vi "sub_APT.vi"() -> ()   [LabVIEW 2015]
panel:
  in  "Up":bool
  in  "Abs. Go":bool
  in  "Down":bool
  in  "Rel Move Size":sgl=1.0 min=-10 max=50 format="%.2f"
  in  "Home Z":bool
  in  "Abs Pos X":sgl=1.0 min=-10 max=360 format="%.2f"
  out "Display Z":sgl(knob) scale=0.0..360.0
  out "Initial Z":bool
  in  "HWSerialNum Z":i32=83856379
  in  "Stop":bool
  in  "MG17Motor Z":refnum<k7>(container)
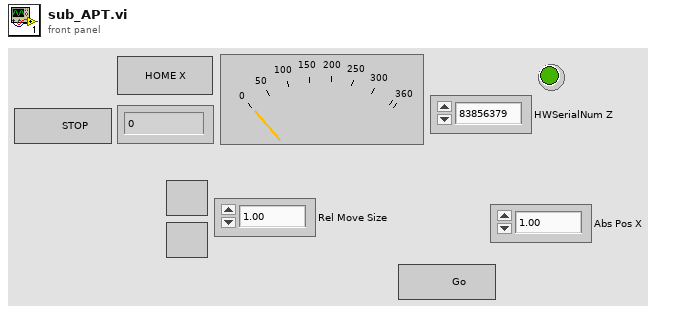
[diagram p1: front panel]
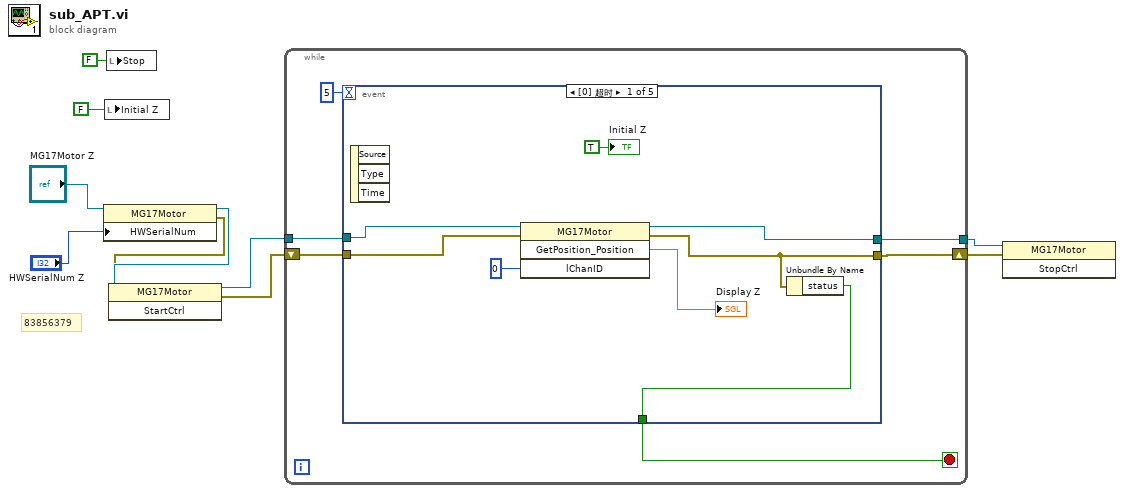
[diagram p0: block diagram]
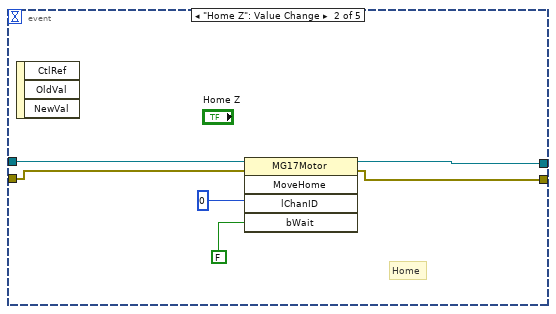
[diagram p2: hidden frame]
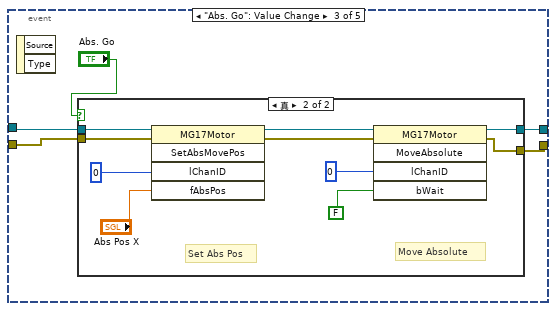
[diagram p3: hidden frame]
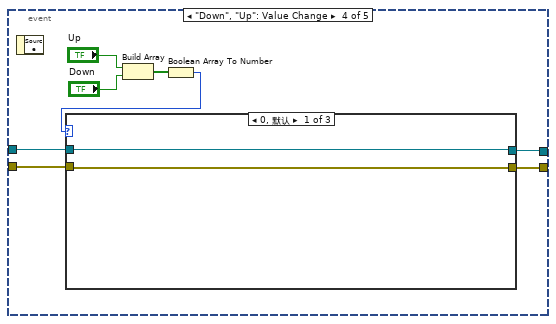
[diagram p5: hidden frame]
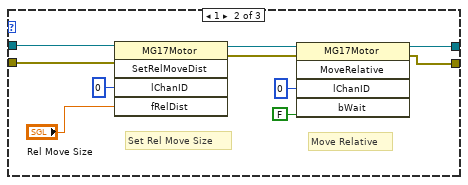
[diagram p6: hidden frame]
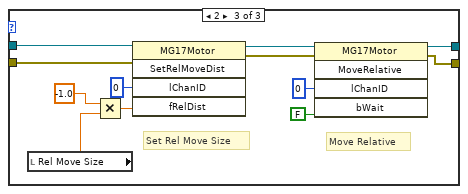
[diagram p7: hidden frame]
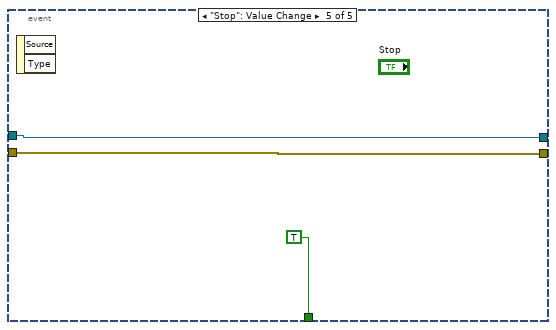
[diagram p8: hidden frame]
diagram:
  # "83856379"
  n1 = property class="MG17Motor"(reference="MG17Motor Z", "HWSerialNum"="HWSerialNum Z") -> (reference out=w9:refnum<k7>, error out=w8:errorcluster)  [unwired: 1 in]
  n2 = local write "Initial Z"(FALSE ("Initial")) -> ()
  n3 = local write "Stop"(FALSE ("Stop")) -> ()
  n4 = invoke class="MG17Motor" method="StartCtrl"(reference=w9, error in=w8) -> (reference out=w7:refnum<k7>, error out=w6:errorcluster)  [unwired: 1 in, 1 out]
  n5 = while {
    shift-right: [w13] -> w4
    shift-left: w6 -> [w15]
    tunnel: w7 -> [w16]
    tunnel: [w14] -> w5
    stop <- w11 stop-if-true
    n6 = event shown="[0] 超时" {
      selector: _ -> [_ _ _ _ _]
      dyn-events: _ -> [_ _ _ _ _]
      timeout: 5 -> [_ _ _ _ _]
      tunnel: w16 -> [w23 w28 w35 w55 w81]
      tunnel: w15 -> [w21 w27 w34 w54 w80]
      tunnel: [w22 w26 w33 w53 w81] -> w14
      tunnel: [w18 w25 w32 w52 w80] -> w13
      tunnel: [w17 _ _ _ TRUE ("Stop")] -> w11
      event Timeout {
        n7 = event-data() -> ()  [unwired: 1 in, 3 out]
        n8 = invoke class="MG17Motor" method="GetPosition_Position"(reference=w23, error in=w21, "lChanID"=0) -> (reference out=w22:refnum<k7>, error out=w18:errorcluster, "GetPosition_Position"=→"Display Z":sgl)  [unwired: 1 in, 1 out]
        n9 = Unbundle By Name(w18) -> ("status"=w17:bool)
        "Initial Z" <- TRUE ("Initial")
      }
      event "Home Z": Value Change {
        # "Home"
        n10 = event-data() -> ()  [unwired: 1 in, 3 out]
        n11 = invoke class="MG17Motor" method="MoveHome"(reference=w28, error in=w27, "lChanID"=0, "bWait"=FALSE) -> (reference out=w26:refnum<k7>, error out=w25:errorcluster)  [unwired: 1 in, 3 out]
      }
      event "Abs. Go": Value Change {
        n12 = event-data() -> ()  [unwired: 1 in, 2 out]
        n13 = case shown="真" "Abs. Go" {
          tunnel: w35 -> [w37 w44]
          tunnel: w34 -> [w36 w43]
          tunnel: [w37 w40] -> w33
          tunnel: [w36 w39] -> w32
          frame False {
          }
          frame True {
            # "Set Abs Pos"
            # "Move Absolute"
            n14 = invoke class="MG17Motor" method="SetAbsMovePos"(reference=w44, error in=w43, "lChanID"=0, "fAbsPos"="Abs Pos X") -> (reference out=w42:refnum<k7>, error out=w41:errorcluster)  [unwired: 1 in, 3 out]
            n15 = invoke class="MG17Motor" method="MoveAbsolute"(reference=w42, error in=w41, "lChanID"=0, "bWait"=FALSE) -> (reference out=w40:refnum<k7>, error out=w39:errorcluster)  [unwired: 1 in, 3 out]
          }
        }
      }
      event "Down", "Up": Value Change {
        n16 = event-data() -> ()  [unwired: 1 in, 1 out]
        n17 = Build Array("Up", "Down") -> (w49:bool[])
        n18 = Boolean Array To Number(Boolean array=w49) -> (number=w48:u32)
        n19 = case shown="0, 默认" w48 {
          tunnel: w55 -> [w57 w62 w74]
          tunnel: w54 -> [w56 w61 w73]
          tunnel: [w57 w60 w72] -> w53
          tunnel: [w56 w59 w71] -> w52
          frame 0, Default {
          }
          frame 1 {
            # "Move Relative"
            # "Set Rel Move Size"
            n20 = invoke class="MG17Motor" method="SetRelMoveDist"(reference=w62, error in=w61, "lChanID"=0, "fRelDist"="Rel Move Size") -> (reference out=w66:refnum<k7>, error out=w67:errorcluster)  [unwired: 1 in, 3 out]
            n21 = invoke class="MG17Motor" method="MoveRelative"(reference=w66, error in=w67, "lChanID"=0, "bWait"=FALSE) -> (reference out=w60:refnum<k7>, error out=w59:errorcluster)  [unwired: 1 in, 3 out]
          }
          frame 2 {
            # "Move Relative"
            # "Set Rel Move Size"
            n22 = local read "Rel Move Size"() -> (w69:sgl)
            n23 = Multiply(x=sgl -1.0, y=w69) -> (x*y=w70:sgl)
            n24 = invoke class="MG17Motor" method="SetRelMoveDist"(reference=w74, error in=w73, "lChanID"=0, "fRelDist"=w70) -> (reference out=w78:refnum<k7>, error out=w79:errorcluster)  [unwired: 1 in, 3 out]
            n25 = invoke class="MG17Motor" method="MoveRelative"(reference=w78, error in=w79, "lChanID"=0, "bWait"=FALSE) -> (reference out=w72:refnum<k7>, error out=w71:errorcluster)  [unwired: 1 in, 3 out]
          }
        }
      }
      event "Stop": Value Change {
        n26 = event-data() -> ()  [unwired: 1 in, 2 out]
      }
    }
  }
  n27 = invoke class="MG17Motor" method="StopCtrl"(reference=w5, error in=w4) -> ()  [unwired: 1 in, 3 out]
